vi "simple_vector_multiply_VI.vi"() -> ()   [LabVIEW 2020]
uses:
  <vilib>/Analysis/baseanly.llb/Vector x A.vi
  <vilib>/Analysis/NI_AALBase.lvlib
panel:
  out "error":dbl
  out "subarray":dbl[](array[numeric])
  out "Array 6":dbl[][](array[numeric])
  out "Array 5":i32[](array[numeric])
  out "Array 4":dbl[](array[numeric])
  out "output array":dbl[](array[numeric])
  out "Array 3":dbl[](array[numeric])
  out "A":dbl[](array[numeric])
  out "V' x A":dbl[](array[numeric])
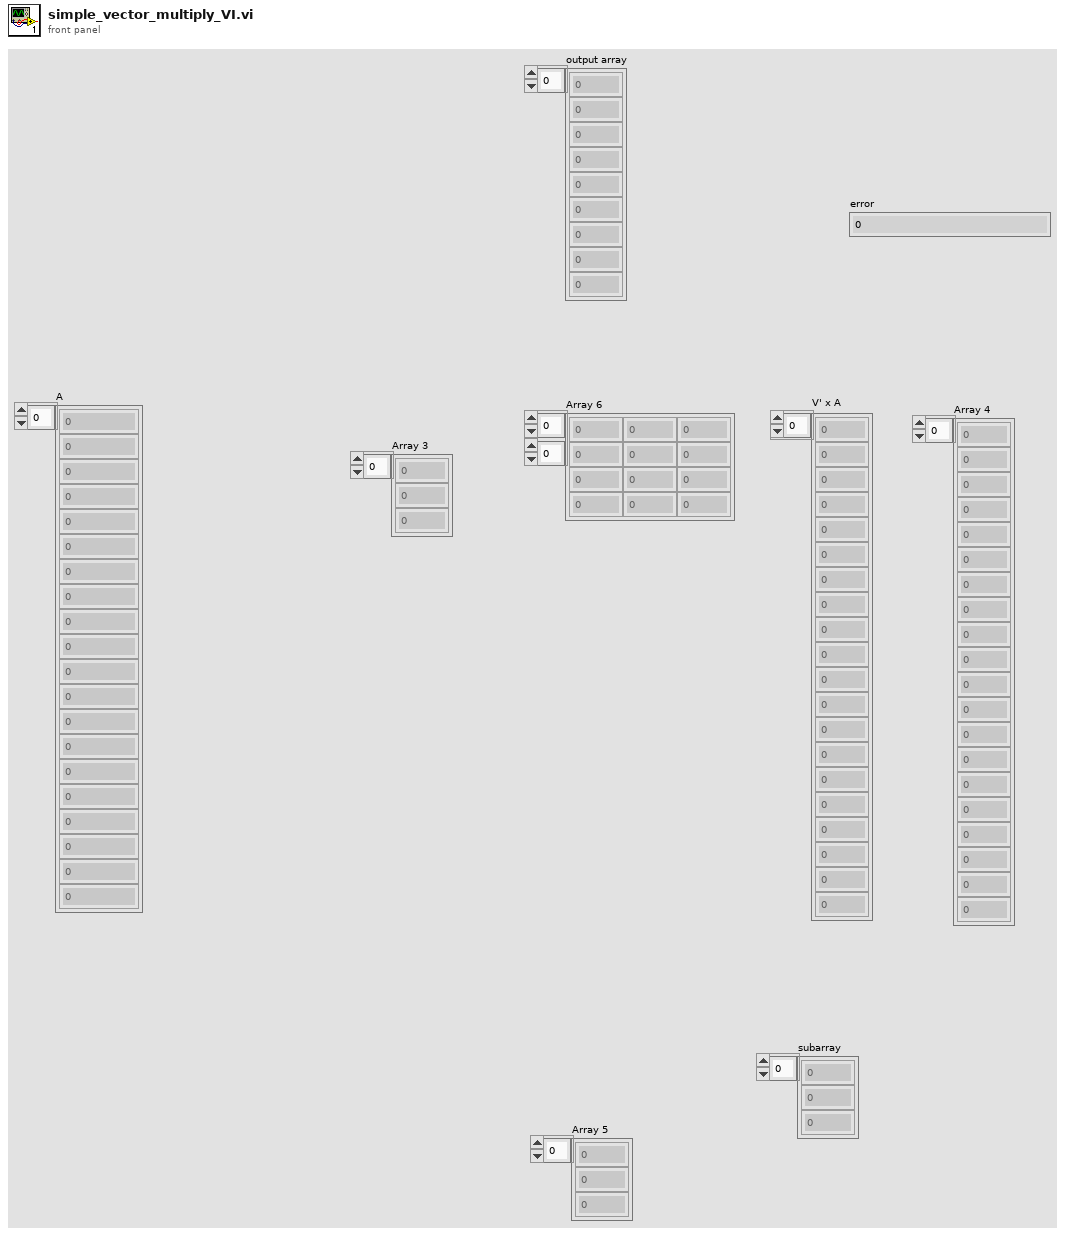
[diagram p1: front panel]
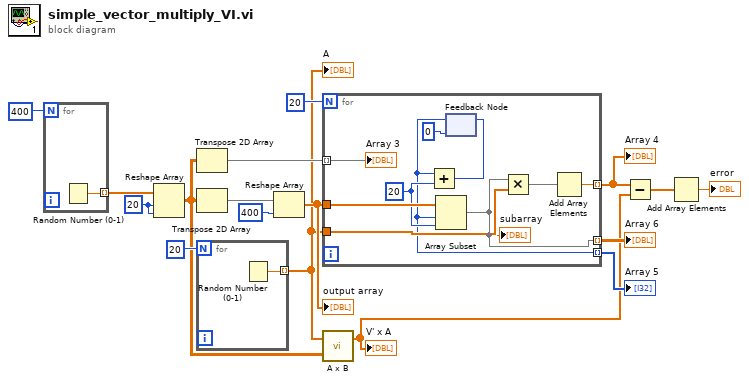
[diagram p0: block diagram]
diagram:
  w3 = 20 ("dimension size")
  n1 = for {
    N: 400 -> [_]
    tunnel: [w18] -> w2 mode=indexing
    n2 = Random Number (0-1)() -> (number: 0 to 1=w18:dbl)
  }
  n3 = Reshape Array(w2, w3, w3) -> (w1:dbl[][])
  n4 = Transpose 2D Array(2D array=w1) -> (transposed array=w16:dbl[][])
  n5 = Transpose 2D Array(2D array=w1) -> (transposed array=w11:dbl[][])
  n6 = for {
    N: 20 -> [_]
    tunnel: [w19] -> w4 mode=indexing
    n7 = Random Number (0-1)() -> (number: 0 to 1=w19:dbl)
  }
  "A" <- w4
  n8 = Reshape Array(w11, 400 ("dimension size")) -> (w14:dbl[])
  "output array" <- w14
  n9 = for {
    N: 20 -> [_]
    tunnel: w16 -> [w29] mode=indexing
    tunnel: w4 -> [w24]
    tunnel: w14 -> [w28]
    tunnel: [w22] -> w10 mode=indexing
    tunnel: [w21] -> w13 mode=indexing
    tunnel: [w20] -> w12 mode=indexing
    w25 = 20 ("length")
    n10 = feedback #1(0) -> (w21:i32)
    n11 = Add(x=w21, y=w25) -> (x+y=w27:i32)
    n12 = Array Subset(array=w28, index=w21, length=w25) -> (w20:dbl[])
    "subarray" <- w20
    n13 = feedback-in #1(w27) -> ()
    n14 = Multiply(x=w20, y=w24) -> (x*y=w23:dbl[])
    n15 = Add Array Elements(numeric array=w23) -> (sum=w22:dbl)
    "Array 3" <- w29
  }
  "Array 4" <- w10
  "Array 5" <- w13
  "Array 6" <- w12
  n16 = call-poly <vilib>:"A x B.vi"("Matrix A"=w1, "Vector V'"=w4) -> ("V' x A"=w9:dbl[])  [unwired: 1 out]
  "V' x A" <- w9
  n17 = Subtract(x=w10, y=w9) -> (x-y=w8:dbl[])
  n18 = Add Array Elements(numeric array=w8) -> (sum=→"error":dbl)
